vi "Find LVClassConstant by Label.vi"(9 "Hide Label? (T)":bool=TRUE, 10 "LabVIEWClassConstant Label":string, 11 "VI Refnum":refnum<vi>) -> (2 "Found?":bool, 3 "Reference":refnum<vi>)   [LabVIEW 2018, in "LVClassByRef.lvlib"]
uses:
  <resource>/Framework/Providers/LVClassByRef/LVClassByRef.lvlib
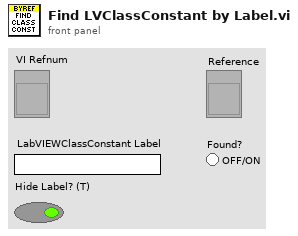
[diagram p1: front panel]
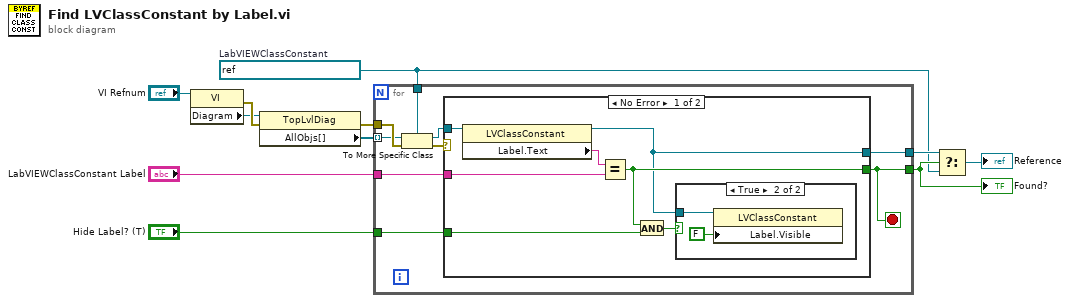
[diagram p0: block diagram]
diagram:
  w2 = refnum<vi> refnum  # LabVIEWClassConstant
  n1 = property class="VI"(reference="VI Refnum") -> (error out=w11:errorcluster, "Diagram"=w10:refnum<vi>)  [unwired: 1 in, 1 out]
  n2 = property class="TopLvlDiag"(reference=w10, error in=w11) -> (error out=w7:errorcluster, "AllObjs[]"=w8:refnum<vi>[])  [unwired: 1 out]
  n3 = for {
    tunnel: w2 -> [w18]
    tunnel: w8 -> [w19] mode=indexing
    tunnel: "LabVIEWClassConstant Label" -> [w15]
    tunnel: "Hide Label? (T)" -> [w14]
    tunnel: [w13] -> w4
    tunnel: w7 -> [w20]
    tunnel: [w12] -> w3
    stop <- w12 stop-if-true
    n4 = To More Specific Class(target class=w18, reference=w19, error in=w20) -> (specific class reference=w16:refnum<vi>, error out=w17:errorcluster)
    n5 = case shown="No Error" w17 {
      tunnel: w16 -> [w27 _]
      tunnel: w15 -> [w25 _]
      tunnel: [w24 _] -> w12
      tunnel: w14 -> [w23 _]
      tunnel: [w21 _] -> w13
      frame No Error {
        n6 = property class="LVClassConstant"(reference=w27) -> (reference out=w21:refnum<vi>, "Label.Text"=w26:string)  [unwired: 1 in, 1 out]
        n7 = Equal?(x=w26, y=w25) -> (x = y?=w24:bool)
        n8 = And(x=w24, y=w23) -> (x .and. y?=w22:bool)
        n9 = case shown="True" w22 {
          tunnel: w21 -> [_ w29]
          frame False {
          }
          frame True {
            n10 = property class="LVClassConstant"(reference=w29, "Label.Visible"=FALSE) -> ()  [unwired: 1 in, 2 out]
          }
        }
      }
      frame Error {
      }
    }
  }
  "Found?" <- w3
  n11 = Select(t=w4, s=w3, f=w2) -> (s? t:f=→"Reference":refnum<vi>)
